vi "Vision - Sections UI.vi"(6 "Local Data in":T2 {"Vision Settings"."Dist/Page" items=["Blue (M)/Black (C)", "Red (M)/Green (C)"]}, 7 "UI Refs":T1, 8 "error in (no error)":errorcluster) -> (0 "error out":errorcluster, 4 "Local Data out":T2 {"Vision Settings"."Dist/Page" items=["Blue (M)/Black (C)", "Red (M)/Green (C)"]})   [LabVIEW 2024]
uses:
  Controls/Vision - Local Data.ctl
  Controls/Test Cluster.ctl
  Controls/Excluded Information.ctl
  Controls/Language.ctl
  Controls/Device_Type.ctl
  <vilib>/Utility/miscctls.llb/LVRectTypeDef.ctl
  <vilib>/Utility/miscctls.llb/LVBoundsTypeDef.ctl
  Controls/Vision - Reporting Settings.ctl
  Controls/Vision - Dist Per Page.ctl
  Controls/Vision - Section.ctl
  Buttons/Bin.ctl
  Controls/Vision - UI Refs.ctl
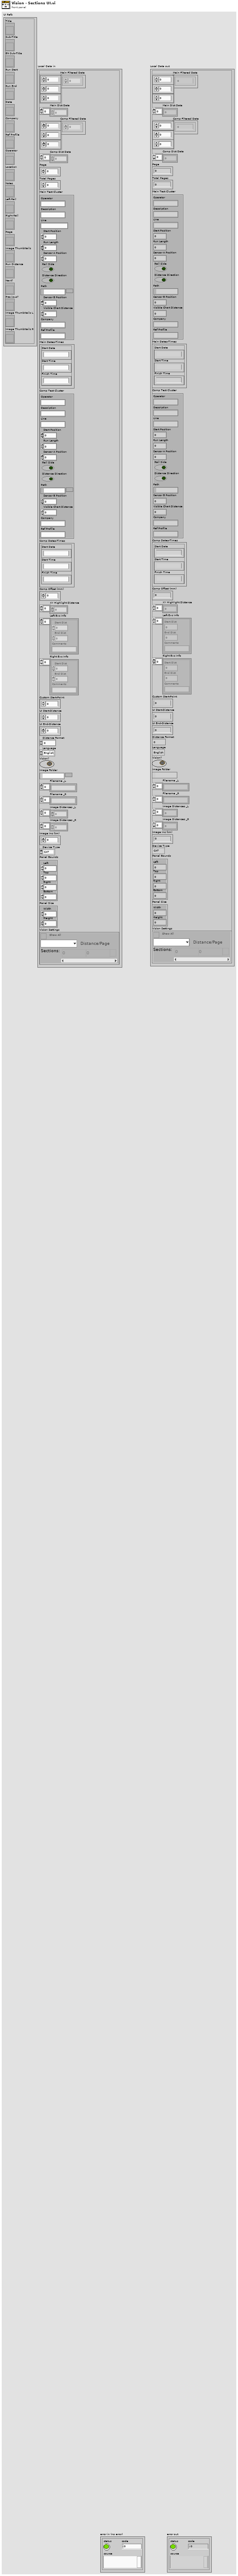
[diagram p1: front panel]
types:
  T1 = typedef "Vision - UI Refs.ctl" = cluster{"Title":refnum<vi>, "Sub-Title":refnum<vi>, "EN Sub-Title":refnum<vi>, "Run Start":refnum<vi>, "Run End":refnum<vi>, "Date":refnum<vi>, "Company":refnum<vi>, "Ref Profile":refnum<vi>, "Operator":refnum<vi>, "Location":refnum<vi>, "Notes":refnum<vi>, "Left Rail":refnum<vi>, "Right Rail":refnum<vi>, "Page":refnum<vi>, "Image ThumbNails":refnum<vi>, "Run Distance":refnum<vi>, "Next?":refnum<vi>, "Previous?":refnum<vi>, "Image ThumbNails L":refnum<vi>, "Image ThumbNails R":refnum<vi>}
  T2 = typedef "Vision - Local Data.ctl" = cluster{"Main Filtered Data":dbl[][][], "Main Dist Data":dbl[], "Comp Filtered Data":dbl[][][], "Comp Dist Data":dbl[], "Page":u8, "Total Pages":u8, "Main Test Cluster":T3, "Main Dates-Times":cluster{"Start Date":string, "Start Time":string, "Finish Time":string}, "Comp Test Cluster":T3, "Comp Dates-Times":cluster{"Start Date":string, "Start Time":string, "Finish Time":string}, "Comp Offset (mm)":i64, "XY Highlight Distance":dbl[], "Left Exc Info":T4[], "Right Exc Info":T4[], "Custom Start-Point":dbl, "UI Start-Distance":dbl, "UI End-Distance":dbl, "Distance Format":u8, "Language":T5, "Vision?":bool, "Image Folder":path, "Filename _L":string[], "Filename _R":string[], "Image Distances _L":dbl[], "Image Distances _R":dbl[], "Image Inc (km)":dbl, "Device Type":T6, "Panel Bounds":T7, "Panel Size":T8, "Vision Settings":T9}
  T3 = typedef "Test Cluster.ctl" = cluster{"Operator":string, "Description":string, "Line":string, "Start Position":dbl, "Run Length":dbl, "Sensor A Position":dbl, "Rail Side":bool, "Distance Direction":bool, "Path":path, "Sensor B Position":dbl, "Visible Chart Distance":dbl, "Company":string, "Ref Profile":string}
  T4 = typedef "Excluded Information.ctl" = cluster{"Start Dist":dbl, "End Dist":dbl, "Comments":string}
  T5 = typedef "Language.ctl" = enum16{"English", "Chinese", "German"}
  T6 = typedef "Device_Type.ctl" = enum16{"CAT", "Bi-CAT", "YRCA", "RCA", "RV-HR", "TV-HR"}
  T7 = typedef "LVRectTypeDef.ctl" = cluster{"Left":i16, "Top":i16, "Right":i16, "Bottom":i16}
  T8 = typedef "LVBoundsTypeDef.ctl" = cluster{"Width":u32, "Height":u32}
  T9 = typedef "Vision - Reporting Settings.ctl" = cluster{"Show All?":bool, "Dist/Page":T10, "Sections":T11[]}
  T10 = typedef "Vision - Dist Per Page.ctl" = u16
  T11 = typedef "Vision - Section.ctl" = cluster{"From":dbl, "To":dbl, "Discard":T12}
  T12 = typedef "Bin.ctl" = bool
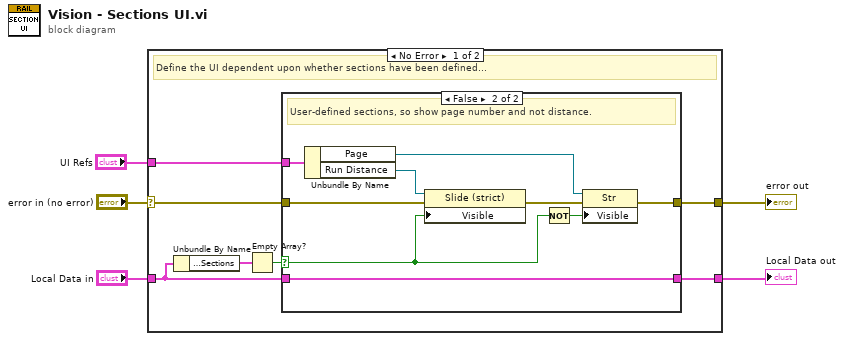
[diagram p0: block diagram]
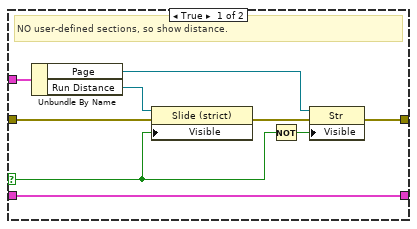
[diagram p2: hidden frame]
diagram:
  n1 = case shown="No Error" "error in (no error)" {
    selector: "error in (no error)" -> [w12 w32]
    tunnel: "Local Data in" -> [w9 w31]
    tunnel: [w10 w31] -> w3
    tunnel: [w11 w32] -> w2
    tunnel: "UI Refs" -> [w6 _]
    frame No Error {
      # "Define the UI dependent upon whether sections have been defined..."
      n2 = Unbundle By Name(w9) -> ("Vision Settings.Sections"=w7:T11[])
      n3 = Empty Array?(array=w7) -> (empty?=w8:bool)
      n4 = case shown="False" w8 {
        selector: w8 -> [w14 w23]
        tunnel: w12 -> [w16 w25]
        tunnel: [w15 w24] -> w11
        tunnel: w9 -> [w21 w30]
        tunnel: [w21 w30] -> w10
        tunnel: w6 -> [w20 w29]
        frame True {
          # "NO user-defined sections, so show distance."
          n5 = Unbundle By Name(w20) -> ("Page"=w18:refnum<vi>, "Run Distance"=w19:refnum<vi>)
          n6 = property class="Slide (strict)"(reference=w19, error in=w16, "Visible"=w14) -> (error out=w17:errorcluster)  [unwired: 1 out]
          n7 = Not(x=w14) -> (.not. x?=w13:bool)
          n8 = property class="Str"(reference=w18, error in=w17, "Visible"=w13) -> (error out=w15:errorcluster)  [unwired: 1 out]
        }
        frame False {
          # "User-defined sections, so show page number and not distance."
          n9 = Unbundle By Name(w29) -> ("Page"=w27:refnum<vi>, "Run Distance"=w28:refnum<vi>)
          n10 = property class="Slide (strict)"(reference=w28, error in=w25, "Visible"=w23) -> (error out=w26:errorcluster)  [unwired: 1 out]
          n11 = Not(x=w23) -> (.not. x?=w22:bool)
          n12 = property class="Str"(reference=w27, error in=w26, "Visible"=w22) -> (error out=w24:errorcluster)  [unwired: 1 out]
        }
      }
    }
    frame Error {
    }
  }
  "error out" <- w2
  "Local Data out" <- w3
